vi "testErrorMessageContainsCustomCaller.vi"() -> ()   [LabVIEW 2019, in "ErrorTest.lvlib" / "ExpectationFailedError.lvlib"]
uses:
  ExpectationFailedError.lvlib
  Error/Error.lvlib
  Assertion/Assertion.lvlib
panel:
  out "error out":errorcluster
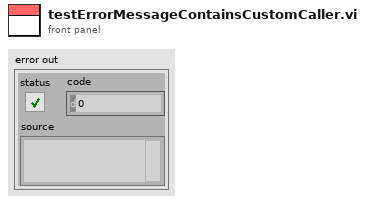
[diagram p1: front panel]
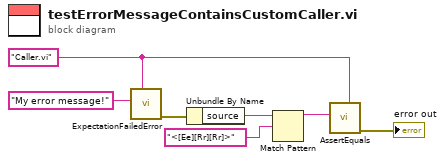
[diagram p0: block diagram]
diagram:
  w1 = "Caller.vi"
  n1 = call "ExpectationFailedError.vi"("Source (caller)"=w1, "Message"="My error message!") -> ("error out"=w5:errorcluster)  [unwired: 9 in]
  n2 = Unbundle By Name(w5) -> ("source"=w4:string)
  n3 = Match Pattern(string=w4, regular expression="<[Ee][Rr][Rr]>") -> (before substring=w2:string)  [unwired: 1 in, 3 out]
  n4 = call "AssertEquals.vi"("Expected"=w1, "Actual"=w2) -> ("error out"=→"error out":errorcluster)  [unwired: 9 in]
